vi "re_msg.incite_lua.vi"(5 "LuaVIEW reference":T1) -> (15 "error out":errorcluster)   [LabVIEW 2012]
doc: "Incite a task to send a reply. This is done by sending the task to be incited a message containing the task identifier of the current task. The incited task can then perform whatever service it is designed to provide and use that identifier to send a reply message when it is done. This function returns on receiving the reply unless an error occurs. BEWARE: when calling this function, you should not be receiving other types of messages at the same time lest these get confused with the incitation reply.\n\nIncitation provides an easy means of synchronously using a service provided by an asynchronous task. More complex message/reply mechanisms can be coded using the messaging primitives. Module export functions also allow a synchronous service to be offered and involve less overhead on account of not requiring a context switch. The advantage of a message/reply mechanism is that the service can be implemented as a task script that can also add asynchronous actions such as periodic updates into the mix. For example:\n\n<pre><code>--#identifier \"myservice\"\nwhile true do\n inciting_task=msg.next()\n if (inciting_task) then\n repeat\n lv.pcall(msg.send,inciting_task,poll(something))\n inciting_task=msg.next()\n until (not inciting_task)\n else\n update(poll(something))\n end\n sleep(update_period)\nend</code></pre>\nParameters:\nstr:task, identifier of the task to incite\n[U32:timeout], timeout in milliseconds. When omitted, the default timeout as specified in the \"incite timeout\" configuration global is used.\nResults:\nstr:reply, reply message\nErrors:\nFunction must be called from a task context but was not.\nTask being incited does not exist or is in error mode.\nTimeout expired before a reply was received."
uses:
  typedefs/t_LuaVIEW Reference.ctl
  subvis/private/LuaVIEW Push (string).vi
  subvis/private/LuaVIEW Pull (string).vi
  subvis/private/LuaVIEW Pull (U32).vi
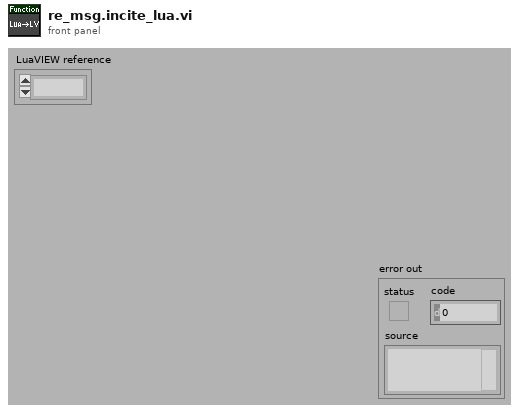
[diagram p1: front panel]
types:
  T1 = typedef "t_LuaVIEW Reference.ctl" = refnum<k1>
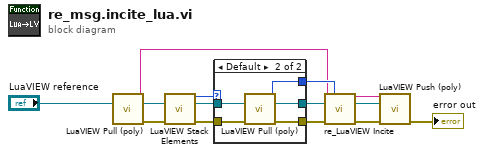
[diagram p0: block diagram]
diagram:
  n1 = call-poly "LuaVIEW Pull (poly).vi"("LuaVIEW reference in"="LuaVIEW reference") -> ("string"=w5:string, "LuaVIEW reference out"=w12:T1, "error out"=w13:errorcluster)  [unwired: 12 in]
  n2 = call "LuaVIEW Stack Elements.vi"("LuaVIEW reference in"=w12, "error in (no error)"=w13) -> ("elements"=w11:i32, "LuaVIEW reference out"=w9:T1, "error out"=w10:errorcluster)  [unwired: 11 in]
  n3 = case shown="Default" w11 {
    tunnel: w10 -> [w16 w21]
    tunnel: w9 -> [w15 w20]
    tunnel: [w16 w19] -> w8
    tunnel: [_ w18] -> w7
    tunnel: [w15 w17] -> w6
    frame 0 {
    }
    frame Default {
      n4 = call-poly "LuaVIEW Pull (poly).vi"("LuaVIEW reference in"=w20, "error in (no error)"=w21) -> ("U32"=w18:u32, "LuaVIEW reference out"=w17:T1, "error out"=w19:errorcluster)  [unwired: 11 in]
    }
  }
  n5 = call "re_LuaVIEW Incite.vi"("task"=w5, "timeout [ms] (use default)"=w7, "LuaVIEW reference in"=w6, "error in (no error)"=w8) -> ("reply"=w3:string, "LuaVIEW reference out"=w2:T1, "error out"=w4:errorcluster)  [unwired: 9 in]
  n6 = call-poly "LuaVIEW Push (poly).vi"("string"=w3, "LuaVIEW reference in"=w2, "error in (no error)"=w4) -> ("error out"=→"error out":errorcluster)  [unwired: 11 in, 1 out]
